vi "TimingFunctions_convertDateStringToTimestamp.vi"(1 "TimeStamp (yymmdd HHMMSS)":string, 5 "error in":errorcluster) -> (15 "TimeStamp (LV)":timestamp, 19 "error out":errorcluster)   [LabVIEW 2016]
doc: "Konvertiert einen String im Format yymmdd HHMMSS in einen Timestamp\n\n15.05.14 / sige"
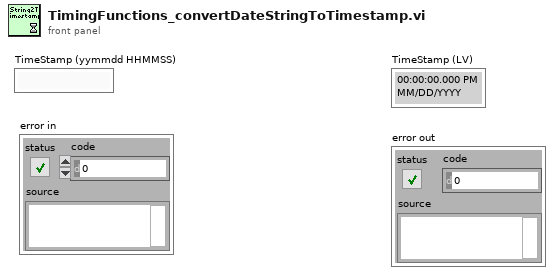
[diagram p1: front panel]
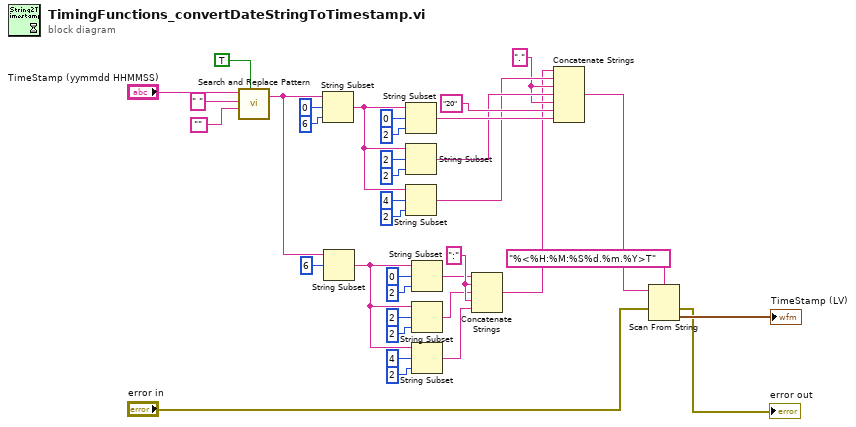
[diagram p0: block diagram]
diagram:
  w13 = ":" ("string")
  w14 = "." ("string")
  n1 = call <vilib>:"Search and Replace Pattern.vi"("string"="TimeStamp (yymmdd HHMMSS)", "regular expression (\"\")"=" " ("regular expression (\"\")"), "replace string (\"\")"="", "replace all? (F)"=TRUE) -> ("result string"=w26:string)  [unwired: 1 in, 1 out]
  n2 = String Subset(string=w26, offset (0)=0, length (rest)=6 ("length (rest)")) -> (substring=w19:string)
  n3 = String Subset(string=w26, offset (0)=6) -> (substring=w6:string)  [unwired: 1 in]
  n4 = String Subset(string=w19, offset (0)=0, length (rest)=2 ("length (rest)")) -> (substring=w18:string)
  n5 = String Subset(string=w19, offset (0)=2, length (rest)=2 ("length (rest)")) -> (substring=w16:string)
  n6 = String Subset(string=w19, offset (0)=4, length (rest)=2 ("length (rest)")) -> (substring=w15:string)
  n7 = String Subset(string=w6, offset (0)=0, length (rest)=2 ("length (rest)")) -> (substring=w5:string)
  n8 = String Subset(string=w6, offset (0)=2, length (rest)=2 ("length (rest)")) -> (substring=w4:string)
  n9 = String Subset(string=w6, offset (0)=4, length (rest)=2 ("length (rest)")) -> (substring=w3:string)
  n10 = Concatenate Strings(w5, w13, w4, w13, w3) -> (w2:string)
  n11 = Concatenate Strings(w2, w15, w14, w16, w14, "20" ("string"), w18) -> (w1:string)
  n12 = Scan From String(format string="%<%H:%M:%S%d.%m.%Y>T", input string=w1, error in="error in") -> (error out=→"error out":errorcluster, output 1=→"TimeStamp (LV)":timestamp)  [unwired: 2 in, 2 out]
